vi "serial_test.vi"() -> ()   [LabVIEW 2015]
uses:
  <vilib>/Instr/_visa.llb/VISA Configure Serial Port (Instr).vi
panel:
  in  "send_btn":bool
  in  "TX":string
  in  "Stop Button":bool
  out "read buffer":string
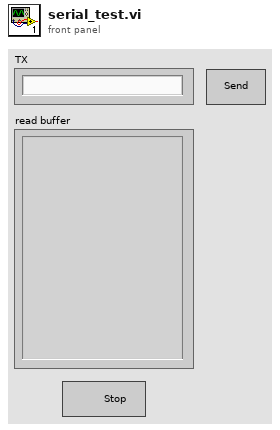
[diagram p1: front panel]
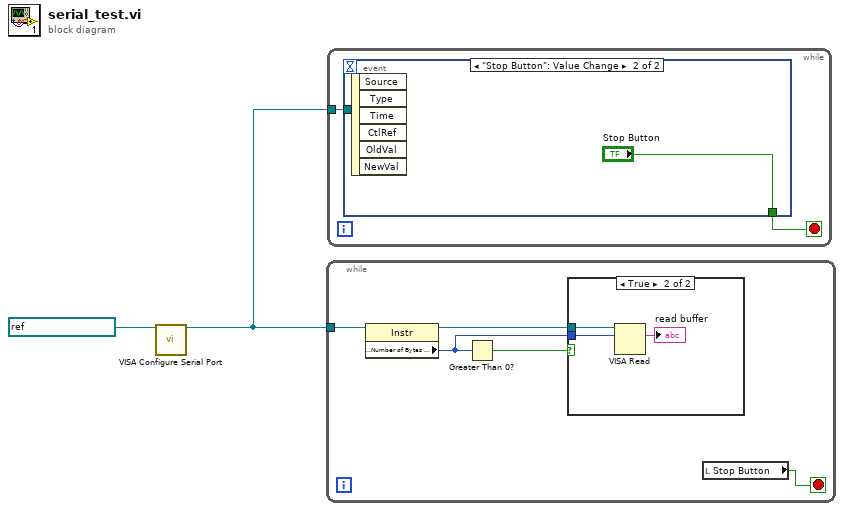
[diagram p0: block diagram]
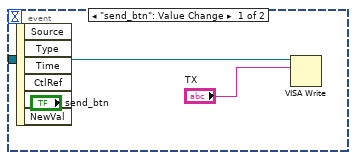
[diagram p2: hidden frame]
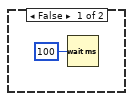
[diagram p3: hidden frame]
diagram:
  n1 = call-poly "VISA Configure Serial Port"("VISA resource name"=refnum<visa-resource-name> "COM4") -> ("VISA resource name out"=w1:refnum<visa-resource-name>)  [unwired: 13 in, 1 out]
  n2 = while {
    tunnel: w1 -> [w7]
    stop <- w3 stop-if-true
    n3 = property class="Instr"(reference=w7) -> (reference out=w4:refnum<visa-resource-name>, "Serial Settings:Number of Bytes at Serial Port"=w5:u32)  [unwired: 1 in, 1 out]
    n4 = Greater Than 0?(x=w5) -> (x > 0?=w6:bool)
    n5 = case shown="True" w6 {
      tunnel: w5 -> [_ w11]
      tunnel: w4 -> [_ w10]
      frame False {
        n6 = Wait (ms)(milliseconds to wait=u32 100) -> ()  [unwired: 1 out]
      }
      frame True {
        n7 = VISA Read(VISA resource name=w10, byte count=w11) -> (read buffer=→"read buffer":string)  [unwired: 1 in, 3 out]
      }
    }
    n8 = local read "Stop Button"() -> (w3:bool)
  }
  n9 = while {
    tunnel: w1 -> [w13]
    stop <- w12 stop-if-true
    n10 = event shown="[1] \"Stop Button\": Value Change" {
      selector: _ -> [_ _]
      dyn-events: _ -> [_ _]
      timeout: _ -> [_ _]
      tunnel: w13 -> [w15 _]
      tunnel: [_ "Stop Button"] -> w12
      event "send_btn": Value Change {
        n11 = event-data() -> ()  [unwired: 1 in, 6 out]
        n12 = VISA Write(VISA resource name=w15, write buffer="TX") -> ()  [unwired: 1 in, 3 out]
      }
      event "Stop Button": Value Change {
        n13 = event-data() -> ()  [unwired: 1 in, 6 out]
      }
    }
  }
